vi "Get Data.vi"(8 "error in":errorcluster, 11 "Alicat Device in":refnum<class "Alicat Device.lvclass">) -> (0 "error out":errorcluster, 2 "Data":refnum<class "Data.lvclass">, 3 "Alicat Device out":refnum<class "Alicat Device.lvclass">)   [LabVIEW 2014, in "Alicat Lib.lvlib" / "Alicat Device.lvclass"]
doc: "Retrieve the data from the Alicat device. The Alicat device takes the address and returns data in a string format in the string <b>DataOut</b>. The data returned is also repackaged into the object <b>Alicat Data</b>."
uses:
  Alicat Device.lvclass
  reusable/Data/Data.lvlibp/Data.lvclass
  Configurable Device/Configurable Device.lvclass/Configurable Device.ctl
  Alicat Device.lvclass/Alicat Device.ctl
  Data/Alicat Data.lvclass/Alicat Data.ctl
  Data/Accessors/Write ID.vi
  Configurable Device/Read ID.vi
  Accessors/Read Alicat Data.vi
  reusable/Session APIs/Serial/Public/Get Data/Get String.vi
  reusable/Data/Data.lvlibp/Write Data ID.vi
  Data/Alicat Data.lvclass
  reusable/Session APIs/Serial/Serial Session.lvclass
panel:
  out "DataOut":string
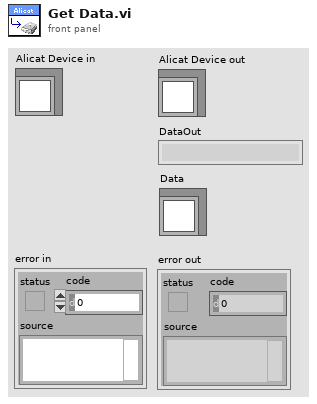
[diagram p1: front panel]
types:
  T1 = typedef "Serial Session.lvclass/Session Handle.ctl" = refnum<data-value>
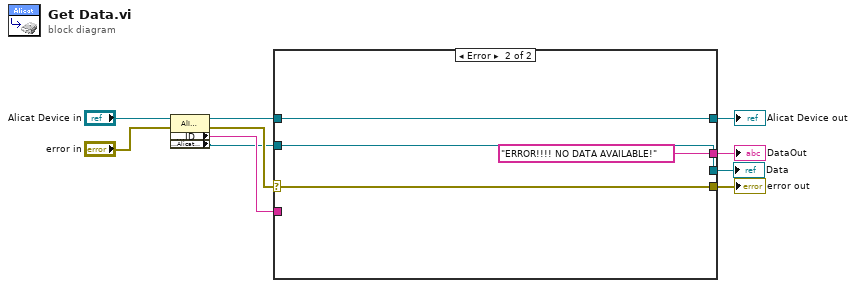
[diagram p0: block diagram]
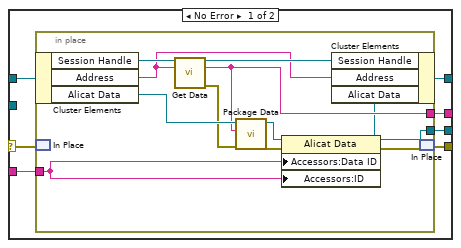
[diagram p2: hidden frame]
diagram:
  n1 = property class="Alicat Device"(reference="Alicat Device in", error in="error in") -> (reference out=w5:refnum<class "Alicat Device.lvclass">, error out=w3:errorcluster, "Accessors:ID"=w2:string, "Accessors:Alicat Data"=w1:refnum<class "Alicat Data.lvclass">)
  n2 = case shown="Error" w3 {
    selector: w3 -> [w16 w32]
    tunnel: w5 -> [w17 w31]
    tunnel: [w14 w32] -> w8
    tunnel: [w15 w31] -> w10
    tunnel: [w13 "ERROR!!!! NO DATA AVAILABLE!" ("DataOut")] -> w9
    tunnel: [w12 w29] -> w7
    tunnel: w2 -> [w11 _]
    tunnel: w1 -> [_ w29]
    frame No Error {
      n3 = in-place {
        in-place-border: [w23] -> w13
        in-place-border: [w18] -> w12
        in-place-border: w11 -> [w22]
        n4 = in-place-cluster #1(w17) -> ("Session Handle"=w28:T1, "Address"=w25:string, "Alicat Data"=w26:refnum<class "Alicat Data.lvclass">)
        n5 = in-place-match #2(w16) -> ()  [unwired: 1 out]
        n6 = call-poly "Get Data.vi"("Session Handle in"=w28, "CMD"=w25) -> ("Session Handle out"=w27:T1, "DataOut"=w23:string, "error out"=w24:errorcluster)  [unwired: 11 in]
        n7 = call-dynamic "Package Data.vi"("error in"=w24, "DataIn"=w23, "Alicat Data in"=w26) -> ("error out"=w20:errorcluster, "Alicat Data out"=w21:refnum<class "Alicat Data.lvclass">)  [unwired: 7 in]
        n8 = property class="Alicat Data"(reference=w21, error in=w20, "Accessors:Data ID"=w22, "Accessors:ID"=w22) -> (reference out=w18:refnum<class "Alicat Data.lvclass">, error out=w19:errorcluster)
        n9 = in-place-cluster #1("Session Handle"=w27, "Address"=w25, "Alicat Data"=w18) -> (w15:refnum<class "Alicat Device.lvclass">)
        n10 = in-place-match #2(w19) -> (w14:errorcluster)
      }
    }
    frame Error {
    }
  }
  "error out" <- w8
  "Alicat Device out" <- w10
  "DataOut" <- w9
  "Data" <- w7
